vi "check if line exists.vi"(8 "error in":errorcluster, 10 "Name to Locate":string, 11 "TDMS datalogger configuration":refnum<class "TDMS datalogger configuration.lvclass">) -> (0 "error out":errorcluster, 1 "Index":i32, 2 "line out":T1, 3 "TDMS datalogger configuration":refnum<class "TDMS datalogger configuration.lvclass">, 5 "Found?":bool)   [LabVIEW 2015, in "TDMS datalogger configuration.lvclass"]
uses:
  TDMS datalogger configuration.lvclass
  <vilib>/NI/Tag Bus Module Framework/channel/TBM channel.lvclass
  TDMS datalogger configuration.lvclass/TDMS datalogger configuration.ctl
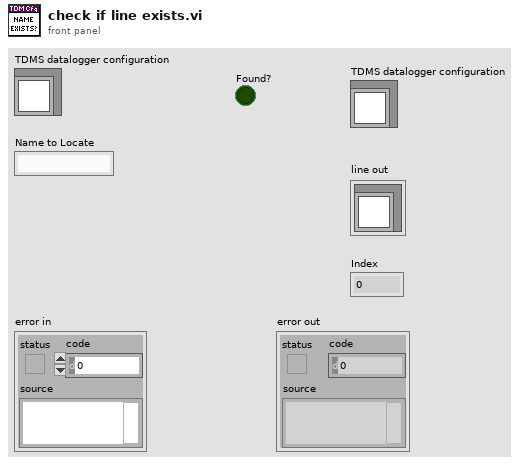
[diagram p1: front panel]
types:
  T1 = cluster{"channel":refnum<class "TBM channel.lvclass">}
  T2 = cluster{"channel":refnum<class "TBM channel.lvclass">}[]
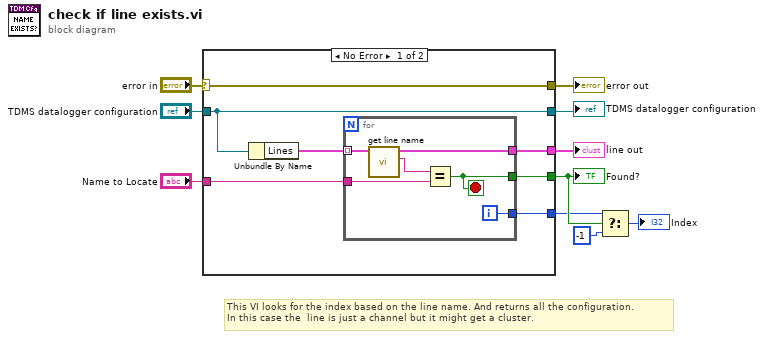
[diagram p0: block diagram]
diagram:
  # "This VI looks for the index based on the line name. And returns all the configuration. \nIn this case the  line is just a channel but it might get a cluster."
  n1 = case shown="No Error" "error in" {
    selector: "error in" -> [w17 w25]
    tunnel: [w17 w25] -> w9
    tunnel: "TDMS datalogger configuration" -> [w12 w24]
    tunnel: "Name to Locate" -> [w15 _]
    tunnel: [w14 _] -> w5
    tunnel: [w13 _] -> w4
    tunnel: [w12 w24] -> w2
    tunnel: [w11 _] -> w1
    frame No Error {
      n2 = Unbundle By Name(w12) -> ("Lines"=w16:T2)
      n3 = for {
        tunnel: w16 -> [w19] mode=indexing
        tunnel: w15 -> [w23]
        tunnel: [w22] -> w14
        tunnel: [w21] -> w13
        tunnel: [w18] -> w11
        i -> [w21]
        stop <- w22 stop-if-true
        n4 = call "get line name.vi"("line in"=w19) -> ("Name"=w20:string, "line out"=w18:T1)  [unwired: 8 in, 1 out]
        n5 = Equal?(x=w20, y=w23) -> (x = y?=w22:bool)
      }
    }
    frame Error {
    }
  }
  "error out" <- w9
  "Found?" <- w5
  "TDMS datalogger configuration" <- w2
  "line out" <- w1
  n6 = Select(t=w4, s=w5, f=-1) -> (s? t:f=→"Index":i32)
